vi "UpdateControlRefnums.vi"(0 "Numeric Refnum":refnum<vi>, 1 "String Refnum":refnum<vi>, 2 "Stop Button Refnum":refnum<vi>, 3 "String To Append":string, 4 "Number of Time To Loop":i32) -> ()   [LabVIEW 2012]
panel:
  out "String":string
  out "Numeric":dbl format="%0.2f"
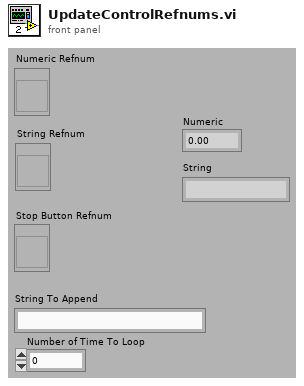
[diagram p1: front panel]
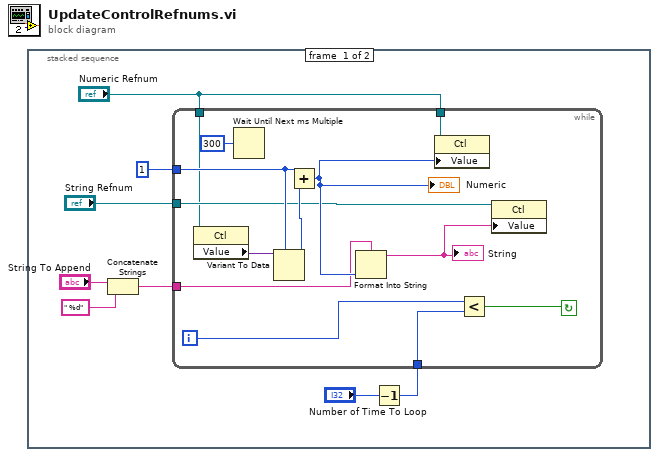
[diagram p0: block diagram]
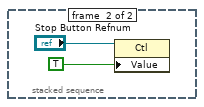
[diagram p2: hidden frame]
diagram:
  n1 = stacked-sequence {
    frame #0 {
      n2 = Concatenate Strings("String To Append", " %d" ("string")) -> (w3:string)
      n3 = Decrement(x="Number of Time To Loop") -> (x-1=w1:i32)
      n4 = while {
        tunnel: 1 ("y") -> [w20]
        tunnel: "Numeric Refnum" -> [w18]
        tunnel: "String Refnum" -> [w15]
        tunnel: "Numeric Refnum" -> [w13]
        tunnel: w3 -> [w10]
        tunnel: w1 -> [w9]
        i -> [w11]
        stop <- w12 continue-if-true
        n5 = property class="Ctl"(reference=w13) -> ("Value"=w14:variant)  [unwired: 1 in, 2 out]
        n6 = Wait Until Next ms Multiple(millisecond multiple=u32 300) -> ()  [unwired: 1 out]
        n7 = Variant To Data(type=w20, Variant=w14) -> (data=w19:i32)  [unwired: 1 in, 1 out]
        n8 = Add(x=w20, y=w19) -> (x+y=w17:i32)
        "Numeric" <- w17
        n9 = Format Into String(format string=w10, w17) -> (resulting string=w16:string)  [unwired: 2 in, 1 out]
        "String" <- w16
        n10 = property class="Ctl"(reference=w18, "Value"=w17) -> ()  [unwired: 1 in, 2 out]
        n11 = Less?(x=w11, y=w9) -> (x < y?=w12:bool)
        n12 = property class="Ctl"(reference=w15, "Value"=w16) -> ()  [unwired: 1 in, 2 out]
      }
    }
    frame #1 {
      n13 = property class="Ctl"(reference="Stop Button Refnum", "Value"=TRUE) -> ()  [unwired: 1 in, 2 out]
    }
  }
